vi "Waveform Replication (RT).vi"() -> ()   [LabVIEW 2023]
doc: "This VI is the VI running on the host PC. This VI starts the controlling VI on FPGA, generates expected waveforms and communicates with the controlling VI on FPGA to read the actual vibration of the shaker and the inverse model of the shaker."
uses:
  <vilib>/rvi/interface/nirviOpenFPGA/nirviOpenFPGA.xnode
  <vilib>/rvi/interface/nirviMethod/nirviMethod.xnode
  <vilib>/rvi/interface/nirviReadWriteControl/nirviReadWriteControl.xnode
  <vilib>/rvi/interface/nirviCloseFPGA/nirviCloseFPGA.xnode
  FPGA Bitfiles/waveformreplicat_FPGATarget_WaveformReplicat_686UJj4wd-w.lvbitx
  Waveform Replication (FPGA).vi
  <vilib>/rvi/errors/niLvFpgaMergeErrorWithErrorCode.vi
  <vilib>/userdefined/High Color/nirio_resource_hc.ctl
panel:
  in  "Tab Control":enum32{"Background", "Road Simulation Control"}(tab)=enum."Road Simulation Control"
  in  "Stop":bool
  in  "Step Size":fxp<+/-,16,-1>=0.05001068115234375
  out "Signals":dbl[](graph)
  out "H(z) - Inverse Model of the Shaker":dbl[](graph)
  in  "Reset":bool
  in  "Delay":i16=500
  in  "Amplitude":dbl=0.1
  in  "Closed Loop":bool
  in  "RIO Device":T1="RIO0"
  # "Waveform replication is to let mechanical or electrical devices replicate an expected waveform exactly. Waveform replication is one of adaptive inverse control applications. Refer to the Adaptive Inverse Control topic in the LabVIEW Help for more information about the background of adaptive inverse control. Select Help>>Show Context Help and move the cursor over the VI icon of this example for more information."
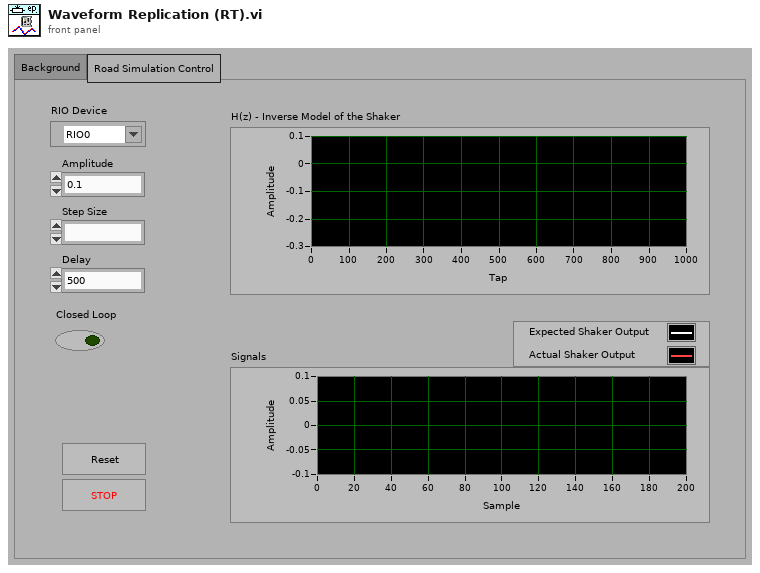
[diagram p1: front panel]
types:
  T1 = typedef "nirio_resource_hc.ctl" = tag
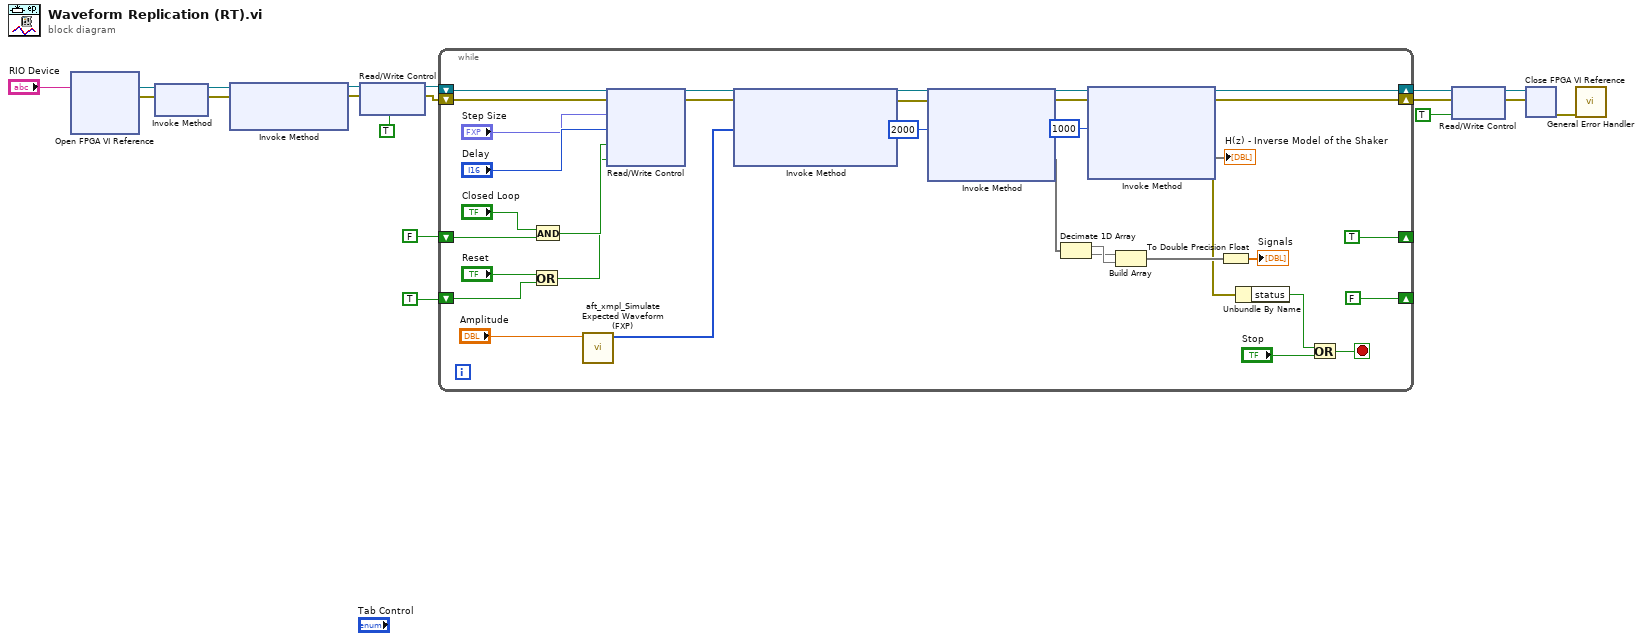
[diagram p0: block diagram]
diagram:
  n1 = xnode "Open FPGA VI Reference"("resource name"="RIO Device") -> ("FPGA VI Reference Out"=w15:refnum<k20>, "error out"=w14:errorcluster)  [unwired: 1 in]
  n2 = xnode "Invoke Method"("FPGA VI Reference In"=w15, "error in"=w14) -> ("FPGA VI Reference Out"=w10:refnum<k20>, "error out"=w9:errorcluster)
  n3 = xnode "Invoke Method"("FPGA VI Reference In"=w10, "error in"=w9) -> ("FPGA VI Reference Out"=w8:refnum<k20>, "error out"=w6:errorcluster)  [unwired: 1 in]
  n4 = xnode "Read/Write Control"("FPGA VI Reference In"=w8, "error in"=w6, "reset? (F)"=TRUE) -> ("FPGA VI Reference Out"=w7:refnum<k20>, "error out"=w5:errorcluster)
  n5 = while {
    shift-right: [w42] -> w12
    shift-left: w7 -> [w50]
    shift-right: [w27] -> w11
    shift-left: w5 -> [w49]
    shift-right: [TRUE] -> _
    shift-left: FALSE -> [w23]
    shift-right: [FALSE] -> _
    shift-left: TRUE -> [w20]
    stop <- w26 stop-if-true
    n6 = Or(x="Reset", y=w20) -> (x .or. y?=w19:bool)
    n7 = And(x="Closed Loop", y=w23) -> (x .and. y?=w37:bool)
    n8 = call "aft_xmpl_Simulate Expected Waveform (FXP).vi"("Amplitude"="Amplitude") -> ("signal"=w30:i32[])  [unwired: 10 out]
    n9 = xnode "Read/Write Control"("FPGA VI Reference In"=w50, "error in"=w49, "step size"="Step Size", "delay"="Delay", "control on?"=w37, "reset? (F)"=w19) -> ("FPGA VI Reference Out"=w48:refnum<k20>, "error out"=w47:errorcluster)
    n10 = xnode "Invoke Method"("FPGA VI Reference In"=w48, "error in"=w47, "Data"=w30) -> ("FPGA VI Reference Out"=w46:refnum<k20>, "error out"=w41:errorcluster)  [unwired: 1 in, 1 out]
    n11 = xnode "Invoke Method"("FPGA VI Reference In"=w46, "error in"=w41, "Number of Elements"=u32 2000) -> ("FPGA VI Reference Out"=w43:refnum<k20>, "Data"=w35:void[])  [unwired: 1 in, 2 out]
    n12 = Decimate 1D Array(w35) -> (w29:void[], w28:void[])
    n13 = xnode "Invoke Method"("FPGA VI Reference In"=w43, "error in"=w41, "Number of Elements"=u32 1000) -> ("FPGA VI Reference Out"=w42:refnum<k20>, "error out"=w27:errorcluster, "Data"=→"H(z) - Inverse Model of the Shaker":void[])  [unwired: 1 in, 1 out]
    n14 = Build Array(w28, w29) -> (w40:void[])
    n15 = To Double Precision Float(number=w40) -> (double precision float=→"Signals":dbl[])
    n16 = Unbundle By Name(w27) -> ("status"=w25:bool)
    n17 = Or(x=w25, y="Stop") -> (x .or. y?=w26:bool)
  }
  n18 = xnode "Read/Write Control"("FPGA VI Reference In"=w12, "error in"=w11, "stop"=TRUE) -> ("FPGA VI Reference Out"=w17:refnum<k20>, "error out"=w16:errorcluster)
  n19 = xnode "Close FPGA VI Reference"("FPGA VI Reference In"=w17, "error in"=w16) -> ("error out"=w1:errorcluster)
  n20 = call <vilib>:"General Error Handler.vi"("error in (no error)"=w1) -> ()  [unwired: 2 in, 13 out]
